vi "Model - Set Amount.vi"(8 "error in (no error)":errorcluster, 10 "Amount":u32, 11 "View Model":T1) -> (0 "error out":errorcluster, 3 "View Model":T1)   [LabVIEW 2017]
doc: "Set actual values of Amount to DVR."
uses:
  Controls/View Model.ctl
  Controls/Shared Model.ctl
  Error Handler/Controls/Error Model.ctl
  Error Handler/Controls/Error Data.ctl
  Error Handler/Controls/Error Type.ctl
  Error Handler/Controls/Error Source.ctl
  Configuration/Controls/Config Model.ctl
  Configuration/Controls/Config CMD.ctl
  Configuration/Controls/Config Command.ctl
  Controller/Controls/Controller Model.ctl
  Controller/Controls/Controller Overhead.ctl
  Controller/Controls/Controller Transaction.ctl
  Controller/Controls/Controller State.ctl
  Configuration/Controls/Config Data Record.ctl
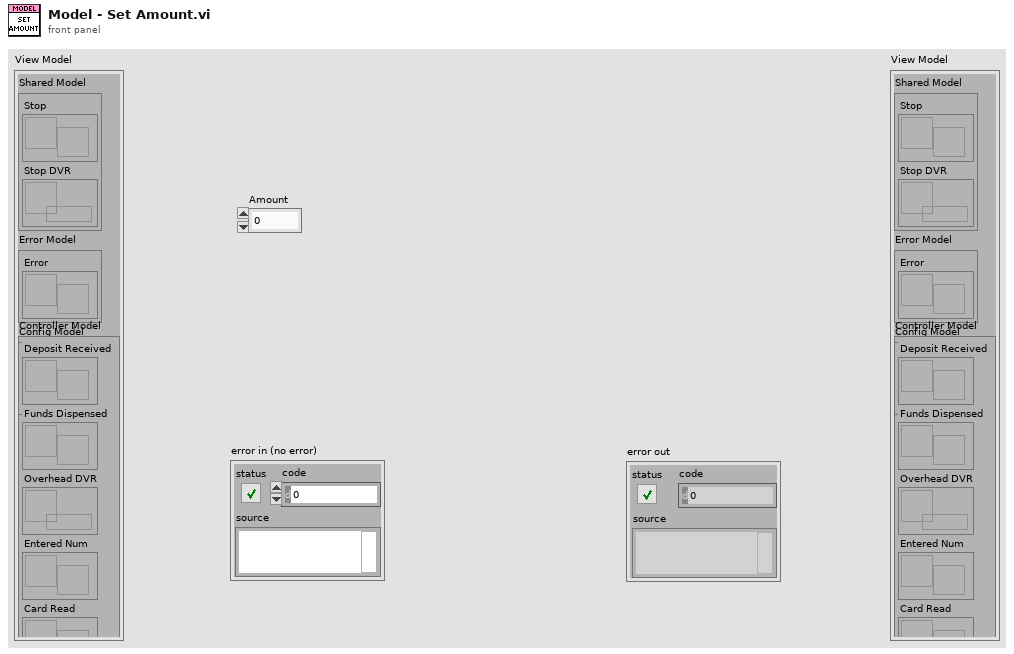
[diagram p1: front panel]
types:
  T1 = typedef "View Model.ctl" = cluster{"Shared Model":T2, "Error Model":T3, "Config Model":T4, "Controller Model":T5}
  T2 = typedef "Shared Model.ctl" = cluster{"Stop":refnum<user-event>, "Stop DVR":refnum<data-value>}
  T3 = typedef "Error Model.ctl" = cluster{"Error":refnum<user-event>}
  T4 = typedef "Config Model.ctl" = cluster{"Config CMD":refnum<user-event>}
  T5 = typedef "Controller Model.ctl" = cluster{"Deposit Received":refnum<user-event>, "Funds Dispensed":refnum<user-event>, "Overhead DVR":refnum<data-value>, "Entered Num":refnum<user-event>, "Card Read":refnum<user-event>, "Transaction":refnum<user-event>}
  T6 = typedef "Controller Overhead.ctl" = cluster{"Account Number":u32, "Amount":u32, "Transaction":T7, "Current State":T8, "Next State":T8, "Elapsed Time":dbl, "User Messages":string[], "Data Record":T9, "Account Found?":bool, "Invalid Login":u8, "Message":string}
  T7 = typedef "Controller Transaction.ctl" = enum16{"Balance Inquiry", "Deposit", "Withdrawal", "Fast Cash", "New Transaction", "Terminate Session"}
  T8 = typedef "Controller State.ctl" = enum16{"Idle", "Initial", "Login", "Balance Inquiry", "Deposit", "Withdrawal", "Fast Cash", "Terminate"}
  T9 = typedef "Config Data Record.ctl" = cluster{"Account Number":u32, "First Name":string, "Last Name":string, "Balance":dbl}
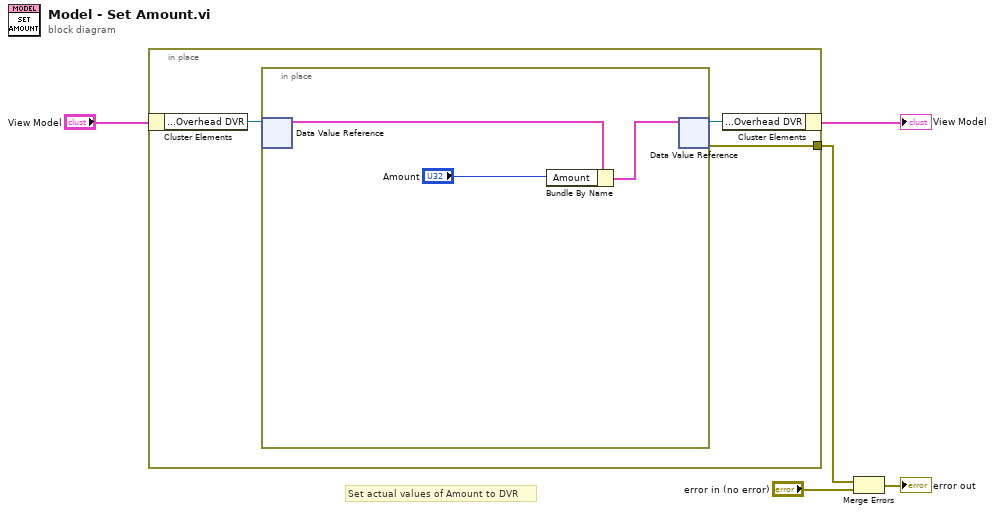
[diagram p0: block diagram]
diagram:
  # "Set actual values of Amount to DVR"
  n1 = in-place {
    in-place-border: [w6] -> w3
    n2 = in-place-cluster #1("View Model") -> ("Controller Model.Overhead DVR"=w8:refnum<data-value>)
    n3 = in-place {
      n4 = in-place-dvr #2(w8) -> (w11:T6)  [unwired: 1 out]
      n5 = Bundle By Name(cluster=w11, "Amount"="Amount") -> (w10:T6)
      n6 = in-place-dvr #2(w10) -> (w7:refnum<data-value>, w6:errorcluster)
    }
    n7 = in-place-cluster #1("Controller Model.Overhead DVR"=w7) -> (→"View Model":T1)
  }
  n8 = Merge Errors(w3, "error in (no error)") -> (→"error out":errorcluster)
